vi "YAV Set Rapidly.vi"() -> ()   [LabVIEW 2018]
doc: "Use this template to build a user interface event handler design pattern. Use this pattern for dialog boxes and other user interfaces. You also can create and execute user-defined events that the VI can handle the same way as user interface events."
uses:
  <instrlib>/Phi6/Common/Instrum/Phi6 Core/YAV-System.llb/YAV Card Total Info.ctl
  <instrlib>/Phi6/Common/Instrum/Phi6 Core/YAV-System.llb/YAV Info.ctl
  <instrlib>/Phi6/Common/Instrum/Phi6 Core/YAV-90132.llb/YAV90132 Type Action.ctl
  <instrlib>/Phi6/Common/Instrum/Phi6 Core/YAV-90132.llb/YAV90132 Mode Action.ctl
  <instrlib>/Phi6/Common/Instrum/Phi6 Core/CANNOU Global Variables.llb/CANNOU Global Variables.gbl.vi
panel:
  out "Cycle":u32
  in  "Info In":T1 {"Version" format="%.0x"; "Options" format="%.0x"; "Index" format="%.0x"}
  in  "stop":bool
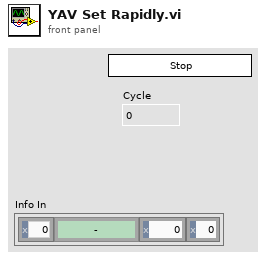
[diagram p1: front panel]
types:
  T1 = typedef "YAV Card Total Info.ctl" = cluster{"Index":u8, "Module":T2, "Version":u16, "Options":u8}
  T2 = typedef "YAV Info.ctl" = enum16{"-", "YAV90832", "YAV904X8", "YAV90132", "YAV91616", "YAV90PIN", "YAV90096", "YAV90HVT", "YAV90CLR", "YAV90128", "YAV90PNE", "YAVCANCON", "YAV91775", "YAV90XXX", "YAV90MMU", "H730050", "H710060", "H710061", "YAV90304", "MMI", "YAV90060", "YAV90MUX", "YAV90059", "YAV90070", "AK087", "Not Defined"}
  T3 = typedef "YAV90132 Type Action.ctl" = enum16{"None", "Set OFF", "Set ON", "TOGGLE", "BLINK", "PULSE ON", "PULSE OFF", "ASK", "Set OUT"}
  T4 = typedef "YAV90132 Mode Action.ctl" = enum16{"None", "One Relay", "Several Relays"}
  T5 = typedef "Module CAN.ctl" = enum16{"CAN0", "CAN1", "CAN2", "CAN3", "CAN4", "CAN5"}
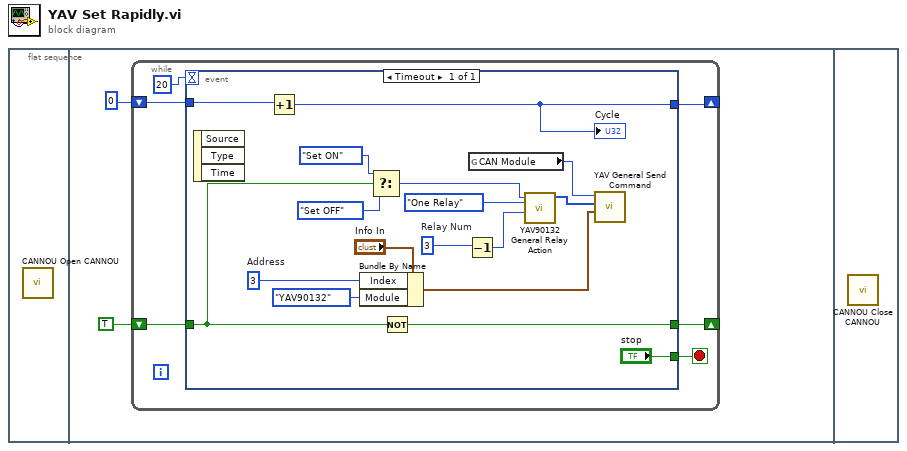
[diagram p0: block diagram]
diagram:
  n1 = flat-sequence {
    frame #0 {
      n2 = call <instrlib>:"CANNOU Open CANNOU.vi"() -> ()  [unwired: 6 in, 2 out]
    }
    frame #1 {
      n3 = while {
        shift-right: [w6] -> _
        shift-left: u32 0 ("x") -> [w7]
        shift-right: [w4] -> _
        shift-left: TRUE ("State") -> [w5]
        stop <- w3 stop-if-true
        n4 = event shown="[0] Timeout" {
          selector: _ -> [_]
          dyn-events: _ -> [_]
          timeout: u32 20 ("x") -> [_]
          tunnel: w7 -> [w13]
          tunnel: [w12] -> w6
          tunnel: w5 -> [w11]
          tunnel: [w10] -> w4
          tunnel: ["stop"] -> w3
          event Timeout {
            w18 = u8 3  # Address
            w19 = u32 3  # Relay Num
            n5 = event-data() -> ()  [unwired: 1 in, 3 out]
            n6 = Increment(x=w13) -> (x+1=w12:u32)
            "Cycle" <- w12
            n7 = Bundle By Name(cluster="Info In", "Index"=w18, "Module"=YAV_Info."YAV90132") -> (w24:T1)
            n8 = Select(t=YAV90132_Type_Action."Set ON" ("Type Action"), s=w11, f=YAV90132_Type_Action."Set OFF") -> (s? t:f=w22:T3)
            n9 = Not(x=w11) -> (.not. x?=w10:bool)
            n10 = Decrement(x=w19) -> (x-1=w25:u32)
            n11 = global read "CANNOU Global Variables.gbl.vi" "CAN Module"() -> (w21:T5)
            n12 = call <instrlib>:"YAV90132 General Relay Action.vi"("Relay/Relays"=w25, "Mode Action"=YAV90132_Mode_Action."One Relay", "Type Action"=w22) -> ("Data"=w23:u8[])  [unwired: 8 in]
            n13 = call <instrlib>:"YAV General Send Command.vi"("Info In"=w24, "Data"=w23, "CAN Module"=w21) -> ()  [unwired: 3 in, 2 out]
          }
        }
      }
    }
    frame #2 {
      n14 = call <instrlib>:"CANNOU Close CANNOU.vi"() -> ()  [unwired: 7 in, 1 out]
    }
  }
